vi "FTW-Logger-FlushToFile.vi"(0 "FTW Logger":refnum<class "FTW-Logger-Core.lvclass">, 11 "error in":errorcluster) -> (4 "FTW Logger out":refnum<class "FTW-Logger-Core.lvclass">, 15 "error out":errorcluster)   [LabVIEW 2013, in "FTW-Logger-Core.lvclass"]
uses:
  FTW-Logger-Core.lvclass
  FTW-Logger-Core.lvclass/FTW-Logger-Core.ctl
panel:
  # "Inputs"
  # "Outputs"
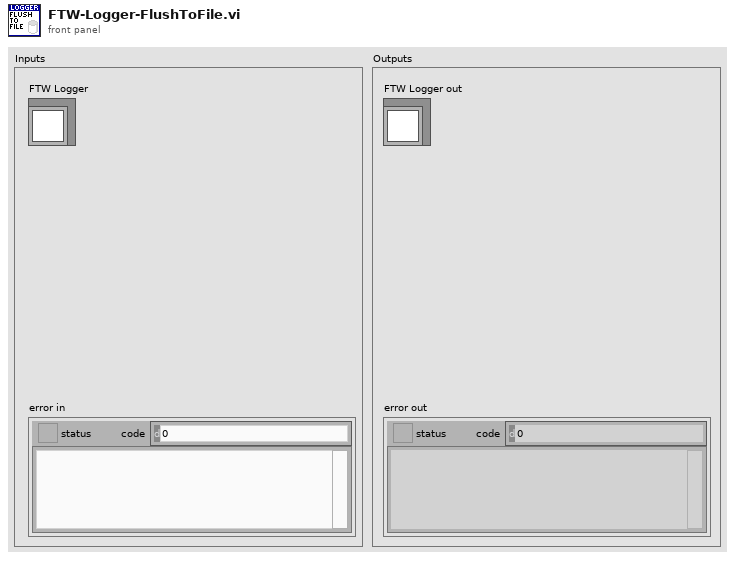
[diagram p1: front panel]
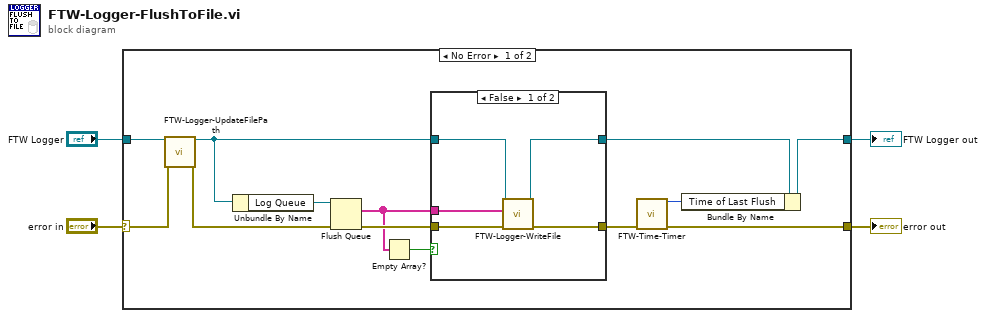
[diagram p0: block diagram]
diagram:
  n1 = case shown="No Error" "error in" {
    selector: "error in" -> [w12 w26]
    tunnel: [w11 w26] -> w1
    tunnel: [w9 w25] -> w3
    tunnel: "FTW Logger" -> [w6 w25]
    frame No Error {
      n2 = call "FTW-Logger-UpdateFilePath.vi"("FTW Logger"=w6, "error in"=w12) -> ("FTW Logger out"=w5:refnum<class "FTW-Logger-Core.lvclass">, "error out"=w7:errorcluster)  [unwired: 12 in]
      n3 = Unbundle By Name(w5) -> ("Log Queue"=w17:refnum<queue>)
      n4 = Flush Queue(queue=w17, error in (no error)=w7) -> (remaining elements=w15:string[], error out=w16:errorcluster)  [unwired: 1 out]
      n5 = Empty Array?(array=w15) -> (empty?=w14:bool)
      n6 = case shown="False" w14 {
        tunnel: [w22 w23] -> w10
        tunnel: w16 -> [w21 w23]
        tunnel: w15 -> [w20 _]
        tunnel: w5 -> [w19 w24]
        tunnel: [w18 w24] -> w13
        frame False {
          n7 = call "FTW-Logger-WriteFile.vi"("FTW Logger"=w19, "Entries to Log"=w20, "error in"=w21) -> ("FTW Logger out"=w18:refnum<class "FTW-Logger-Core.lvclass">, "error out"=w22:errorcluster)  [unwired: 11 in]
        }
        frame True {
        }
      }
      n8 = call "FTW-Time-Timer.vi"("error in"=w10) -> ("Current Tick Count"=w8:u32, "error out"=w11:errorcluster)  [unwired: 12 in, 1 out]
      n9 = Bundle By Name(cluster=w13, "Time of Last Flush"=w8) -> (w9:refnum<class "FTW-Logger-Core.lvclass">)
    }
    frame Error {
    }
  }
  "error out" <- w1
  "FTW Logger out" <- w3
